vi "LabVIEW Image Size.vi"(0 "Cluster":T1) -> (1 "Width":i16, 2 "Height":i16)   [LabVIEW 2011, in "labvvis.lvlib"]
doc: "Returns the width and height of a LabVIEW image."
uses:
  <userlib>/labvvis/labvvis.lvlib
  <vilib>/picture/picture.llb/imagedata.ctl
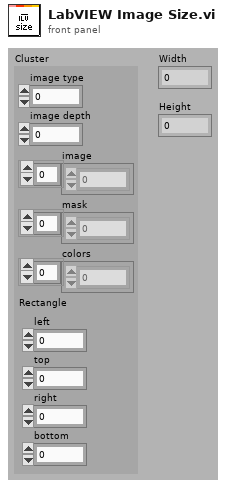
[diagram p1: front panel]
types:
  T1 = typedef "imagedata.ctl" = cluster{"image type":i32, "image depth":i32, "image":u8[], "mask":u8[], "colors":u32[], "Rectangle":cluster{"left":i16, "top":i16, "right":i16, "bottom":i16}}
  T2 = cluster{"left":i16, "top":i16, "right":i16, "bottom":i16}
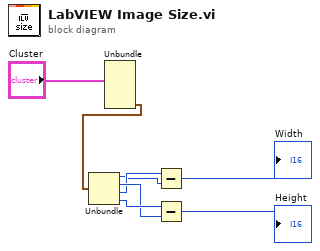
[diagram p0: block diagram]
diagram:
  n1 = Unbundle("Cluster") -> ("Rectangle"=w3:T2)  [unwired: 5 out]
  n2 = Unbundle(w3) -> ("left"=w5:i16, "top"=w7:i16, "right"=w6:i16, "bottom"=w8:i16)
  n3 = Subtract(x=w6, y=w5) -> (x-y=→"Width":i16)
  n4 = Subtract(x=w8, y=w7) -> (x-y=→"Height":i16)
